vi "Read TCP.vi"(8 "error in (no error)":errorcluster, 9 "Timeout (ms)":i32, 10 "Bytes to Read":i32=1, 11 "LiDAR in":refnum<class "LiDAR.lvclass">) -> (0 "error out":errorcluster, 2 "Data Out":string, 3 "LiDAR out":refnum<class "LiDAR.lvclass">)   [LabVIEW 2018, in "LiDAR.lvlib" / "LiDAR.lvclass"]
uses:
  LiDAR.lvclass
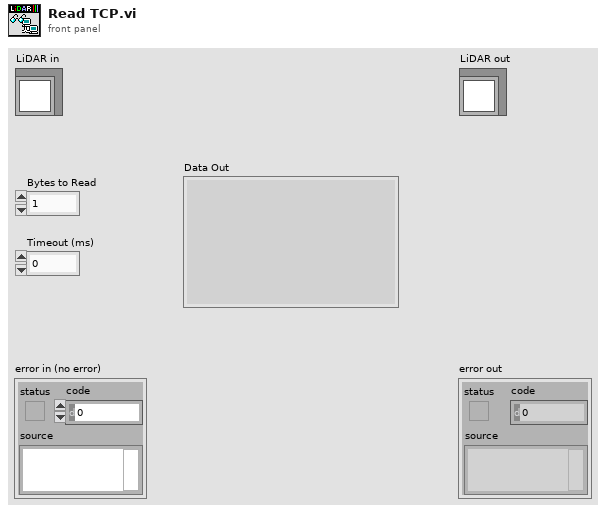
[diagram p1: front panel]
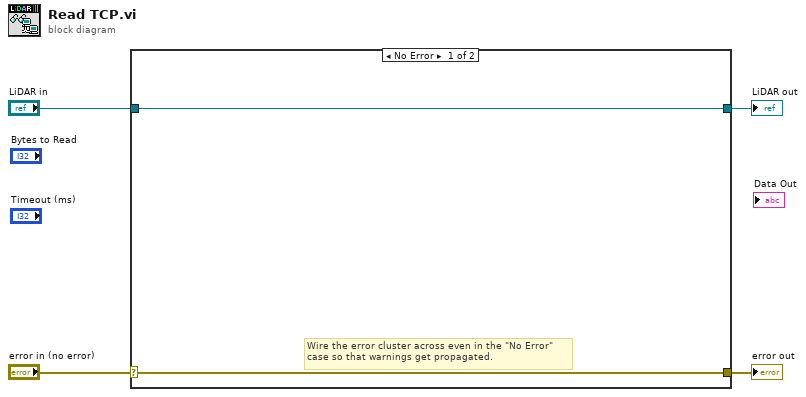
[diagram p0: block diagram]
diagram:
  n1 = case shown="No Error" "error in (no error)" {
    selector: "error in (no error)" -> [w5 w8]
    tunnel: [w5 w8] -> w3
    tunnel: [w6 w7] -> w1
    tunnel: "LiDAR in" -> [w6 w7]
    frame No Error {
      # "Wire the error cluster across even in the \"No Error\"\ncase so that warnings get propagated."
    }
    frame Error {
    }
  }
  "error out" <- w3
  "LiDAR out" <- w1
